vi "SPCM_DLL_path.vi"() -> ()   [LabVIEW 2012]
panel:
  out "DLL loaded":bool=TRUE
  in  "DLL_path":path=path "C:/Program Files (x86)/BH/SPCM/DLL/spcm64.dll"
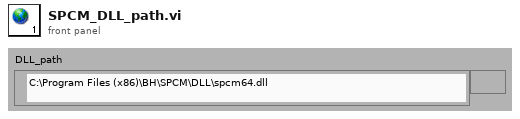
[diagram p1: front panel]
diagram:
